vi "Merge Patch ATTEMPT 1.vi"(4 "null means delete (T)":bool=TRUE, 6 "Item Name":string, 7 "Object (or Item) Path":string, 8 "error in (no error)":errorcluster, 9 "JSON Patch":string, 10 "Object Offset":i32, 11 "JSON in":string="{}") -> (0 "error out":errorcluster, 3 "<JSON>":string)   [LabVIEW 2015, in "JSONtext.lvlib"]
doc: "Insert JSON item at the Path specified."
uses:
  JSONtext.lvlib
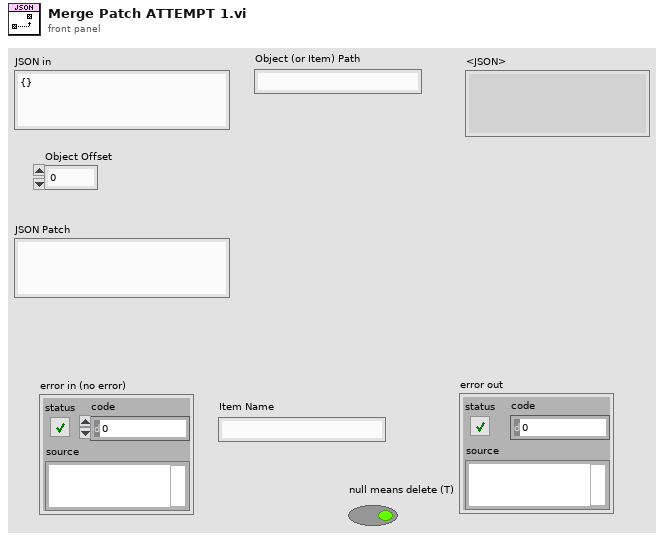
[diagram p1: front panel]
types:
  T1 = typedef "JSONtext.lvlib/Found Items.ctl" = cluster{"Item offset":i32, "Offset past Item":i32, "Name offset":i32, "Offset past Name":i32, "Found":bool, "Item Type":T2, "Item Index":i32}
  T2 = typedef "JSONtext.lvlib/Parsing State.ctl" = enum16{"Parser Error", "Object", "Array", "String", "Number/Other", "Leading Whitespace", "Object end", "Array end", "Value end"}
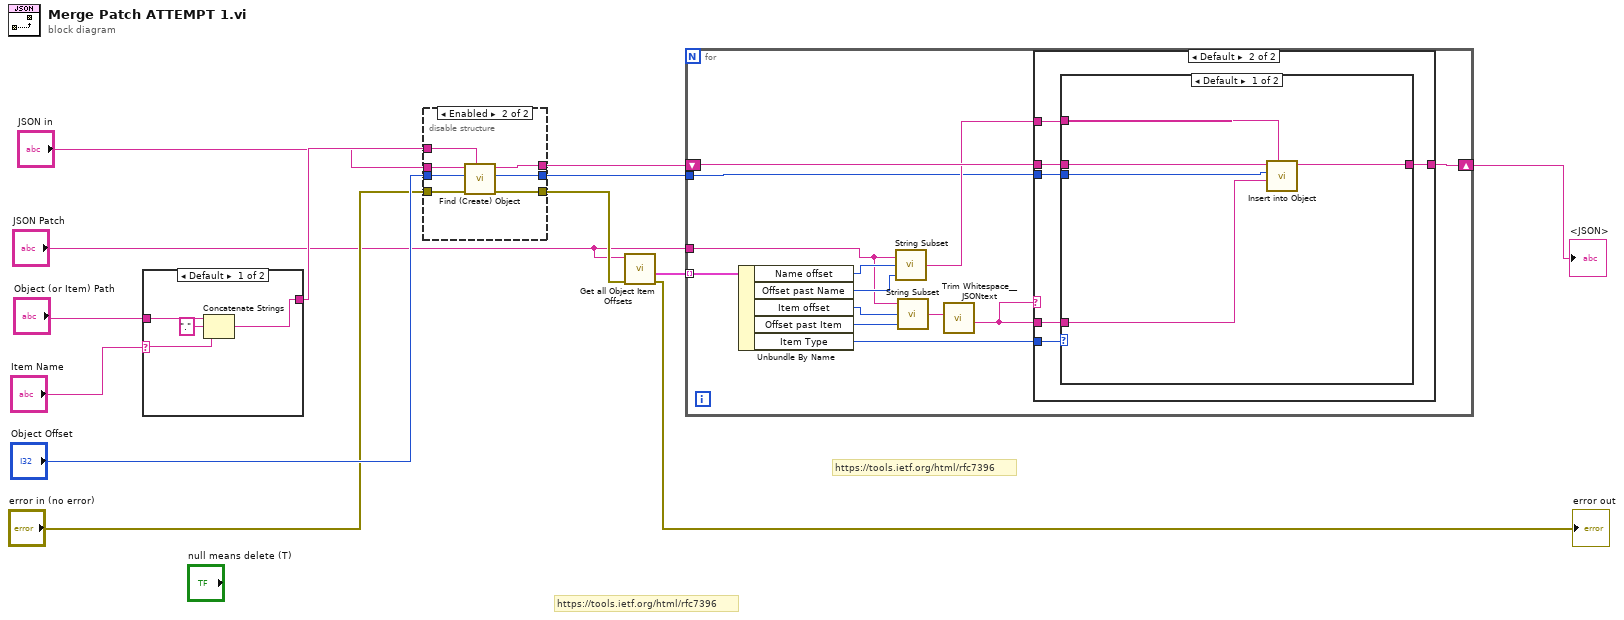
[diagram p0: block diagram]
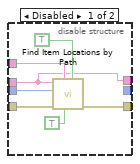
[diagram p2: hidden frame]
diagram:
  # "https://tools.ietf.org/html/rfc7396"
  # "https://tools.ietf.org/html/rfc7396"
  n1 = case shown="Default" "Item Name" {
    selector: "Item Name" -> [w14 _]
    tunnel: "Object (or Item) Path" -> [w17 w18]
    tunnel: [w15 w18] -> w7
    frame Default {
      n2 = Concatenate Strings(w17, "." ("string"), w14) -> (w15:string)
    }
    frame "" {
    }
  }
  n3 = disable-structure shown="Enabled" {
    disable-tunnel: "Object Offset" -> [w25 w29]
    disable-tunnel: "error in (no error)" -> [w22 w30]
    disable-tunnel: [w21 w28] -> w9
    disable-tunnel: w7 -> [w20 w31]
    disable-tunnel: "JSON in" -> [w19 w32]
    disable-tunnel: [w19 w27] -> w4
    disable-tunnel: [_ w26] -> w3
    frame Disabled {
      n4 = call "Find Item Locations by Path.vi"("Insertion point if not found"=TRUE, "Only return first found"=TRUE, "Path"=w20, "error in (no error)"=w22, "Object Offset"=w25, "JSON"=w19) -> ("error out"=w21:errorcluster)  [unwired: 4 in, 1 out]
    }
    frame Enabled {
      n5 = call "Find (Create) Object.vi"("Object Path"=w31, "error in (no error)"=w30, "Starting Offset"=w29, "JSON"=w32) -> ("error out"=w28:errorcluster, "Object offset"=w26:i32, "<JSON>"=w27:string)  [unwired: 5 in]
    }
  }
  n6 = call "Get all Object Item Offsets.vi"("error in (no error)"=w9, "JSON"="JSON Patch") -> ("error out"=→"error out":errorcluster, "Items"=w8:T1[])  [unwired: 7 in, 1 out]
  n7 = for {
    tunnel: w8 -> [w45] mode=indexing
    tunnel: "JSON Patch" -> [w42]
    tunnel: w3 -> [w34]
    shift-right: [w33] -> w2
    shift-left: w4 -> [w39]
    n8 = Unbundle By Name(w45) -> ("Name offset"=w44:i32, "Offset past Name"=w43:i32, "Item offset"=w41:i32, "Offset past Item"=w40:i32, "Item Type"=w35:T2)
    n9 = call "String Subset.vi"("Offset past End"=w43, "Start offset"=w44, "JSON"=w42) -> ("substring"=w38:string)  [unwired: 2 in]
    n10 = call "String Subset.vi"("Offset past End"=w40, "Start offset"=w41, "JSON"=w42) -> ("substring"=w37:string)  [unwired: 2 in]
    n11 = call "Trim Whitespace__JSONtext.vi"("String in"=w37) -> ("String out"=w36:string)  [unwired: 6 in]
    n12 = case shown="Default" w36 {
      tunnel: w39 -> [w46 w49]
      tunnel: w38 -> [_ w51]
      tunnel: w36 -> [_ w50]
      tunnel: w35 -> [_ w52]
      tunnel: w34 -> [_ w48]
      tunnel: [w46 w47] -> w33
      frame "null" {
        # "Delete"
      }
      frame Default {
        n13 = case shown="Default" w52 {
          tunnel: w51 -> [w56 _]
          tunnel: w50 -> [w55 _]
          tunnel: w49 -> [w57 w58]
          tunnel: w48 -> [w54 _]
          tunnel: [w53 w58] -> w47
          frame Default {
            n14 = call "Insert into Object.vi"("Object (or Item) Path"=w56, "JSON to Insert"=w55, "Object Offset"=w54, "JSON in"=w57) -> ("<JSON>"=w53:string)  [unwired: 4 in, 2 out]
          }
          frame "Object" {
          }
        }
      }
    }
  }
  "<JSON>" <- w2
